vi "OddOrEven.vi"(0 "Value":dbl) -> (1 "Is even?":bool, 2 "Is odd?":bool, 3 "Is fractional?":bool)   [LabVIEW 2011]
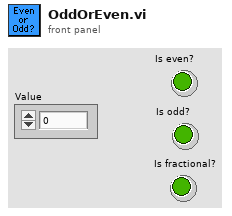
[diagram p1: front panel]
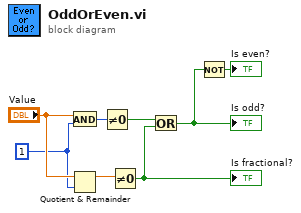
[diagram p0: block diagram]
diagram:
  w4 = 1 ("y")
  n1 = And(x="Value", y=w4) -> (x .and. y?=w8:i32)
  n2 = Quotient & Remainder(x="Value", y=w4) -> (x-y*floor(x/y)=w3:dbl)  [unwired: 1 out]
  n3 = Not Equal To 0?(x=w8) -> (x != 0?=w7:bool)
  n4 = Not Equal To 0?(x=w3) -> (x != 0?=w1:bool)
  "Is fractional?" <- w1
  n5 = Or(x=w7, y=w1) -> (x .or. y?=w2:bool)
  "Is odd?" <- w2
  n6 = Not(x=w2) -> (.not. x?=→"Is even?":bool)
